vi "main.vi"(11 "Message Input":T1) -> (5 "Message Output":T1)   [LabVIEW 2025, in "Module 2.lvlib"]
uses:
  Module 2.lvlib
  <extravilib>/ChannelInstances/Event Messenger-t'Channel Messages.lvlib-Message Cluster.ctl'/))Channel.ctl
  Channel Messages/Message Cluster.ctl
  Module 2 Cases.ctl
  0fcfb8a4-f357-4310-b837-e68650746e25.vi
  <vilib>/Utility/error.llb/Clear Errors.vi
  <extravilib>/ChannelInstances/Event Messenger-t'Channel Messages.lvlib-Message Cluster.ctl'/))Channel.vi
  Channel Messages/9242 error converting cmd string to case enum--error.vi
  <extravilib>/ChannelInstances/Event Messenger-t'Channel Messages.lvlib-Message Cluster.ctl'.lvlib
  Channel Messages/Channel Messages.lvlib
panel:
  in  "Process Stop Button":bool
  in  "Record Button":bool
  out "Log":string
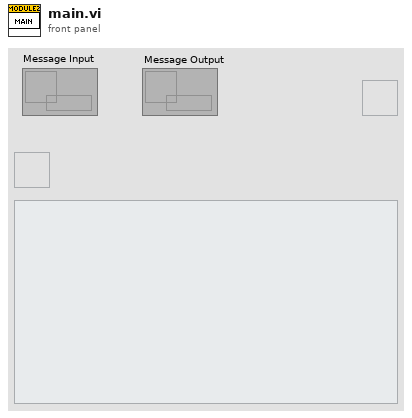
[diagram p1: front panel]
types:
  T1 = typedef "Event Messenger-t'Channel Messages.lvlib-Message Cluster.ctl'.lvlib/))Channel.ctl" = refnum<queue>
  T2 = typedef "Channel Messages.lvlib/Message Cluster.ctl" = cluster{"cmd":string, "data":variant}
  T3 = typedef "Module 2 Cases.ctl" = enum16{"Kill", "Stop", "Start", "Log"}
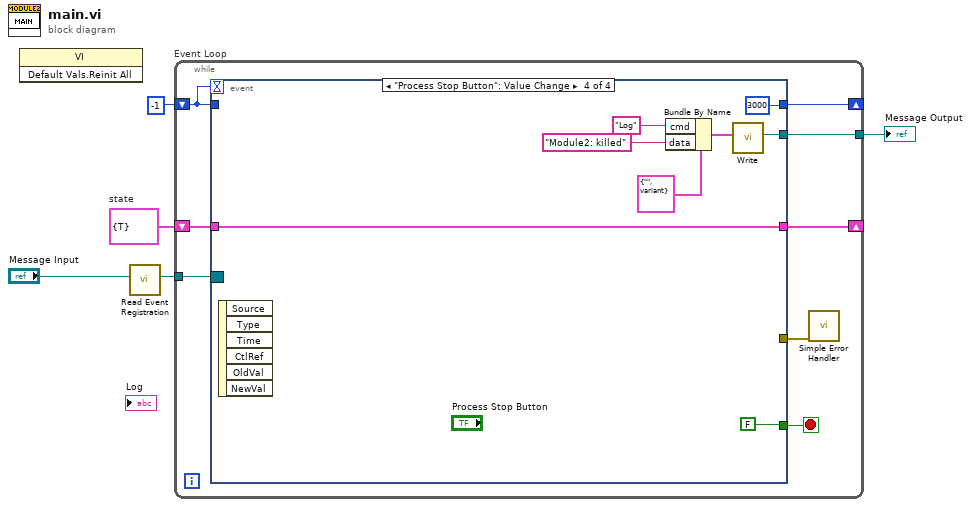
[diagram p0: block diagram]
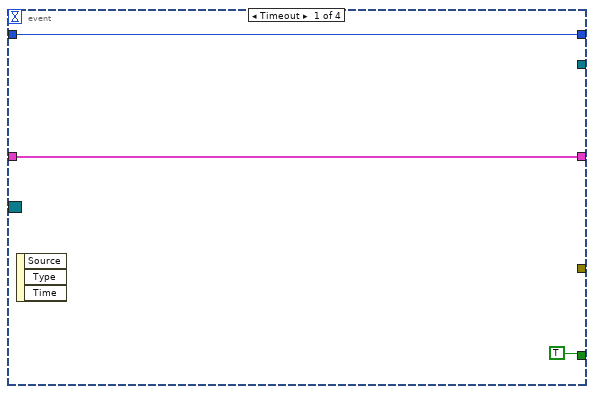
[diagram p2: hidden frame]
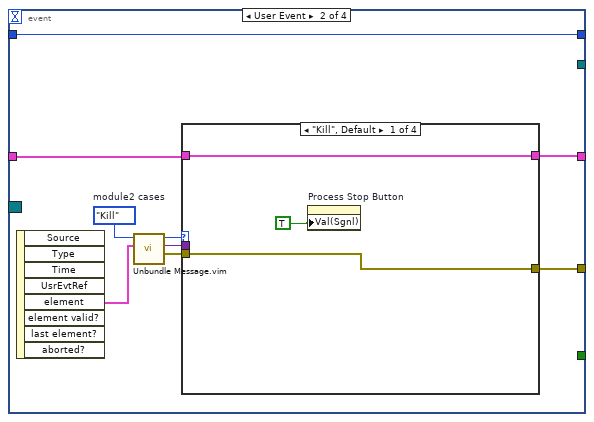
[diagram p3: hidden frame]
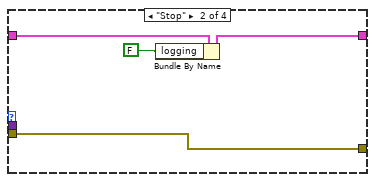
[diagram p4: hidden frame]
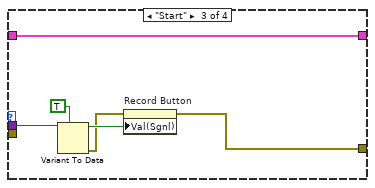
[diagram p5: hidden frame]
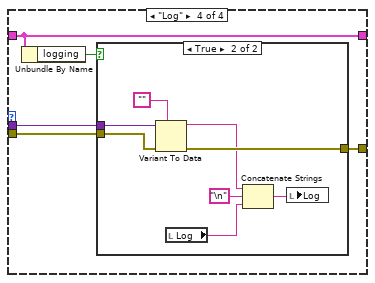
[diagram p6: hidden frame]
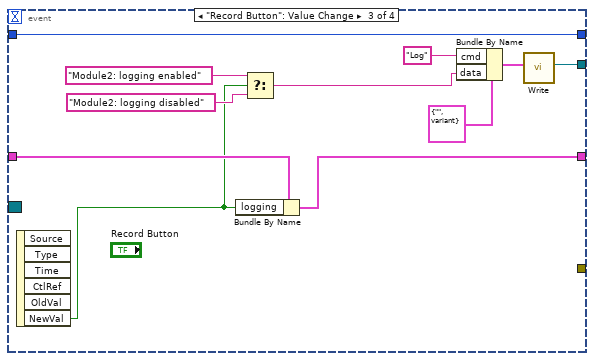
[diagram p8: hidden frame]
diagram:
  w5 = cluster{"logging":bool} {"logging"=TRUE}  # state
  n1 = invoke class="VI" method="Default Vals.Reinit All"() -> ()  [unwired: 3 in, 3 out]
  n2 = call <extravilib>:"Read Event Registration.vi"("channel"="Message Input") -> ("event registration refnum"=w3:refnum<event-registration>)  [unwired: 10 in]
  n3 = while "Event Loop" {
    shift-right: [w11] -> _
    shift-left: w5 -> [w12]
    tunnel: w3 -> [w9]
    tunnel: [w8] -> w2
    shift-right: [w6] -> _
    shift-left: -1 -> [w7]
    stop <- w13 stop-if-true
    n4 = event shown="[3] \"Process Stop Button\": Value Change" {
      selector: w9 -> [_ _ _ _]
      dyn-events: _ -> [_ _ _ _]
      timeout: w7 -> [_ _ _ _]
      tunnel: [TRUE _ _ FALSE] -> w13
      tunnel: w12 -> [w14 w22 w63 w64]
      tunnel: [w14 w21 w62 w64] -> w11
      tunnel: [_ w19 _ _] -> w10
      tunnel: [_ _ w57 w68] -> w8
      tunnel: w7 -> [w15 w17 w53 _]
      tunnel: [w15 w17 w53 3000] -> w6
      event Timeout {
        n5 = event-data() -> ()  [unwired: 1 in, 3 out]
      }
      event User Event {
        w24 = Module_2_Cases."Kill"  # module2 cases
        n6 = event-data() -> ("element"=w23:T2)  [unwired: 1 in, 7 out]
        n7 = call "Unbundle Message.vim"("message"=w23, "cases type"=w24) -> ("error out"=w20:errorcluster, "data"=w25:variant, "case"=w18:T3)  [unwired: 7 in]
        n8 = case shown="\"Kill\", Default" w18 {
          tunnel: w25 -> [_ _ w38 w41]
          tunnel: w22 -> [w28 w32 w33 w43]
          tunnel: [w28 w30 w33 w43] -> w21
          tunnel: [w27 w31 w34 w40] -> w19
          tunnel: w20 -> [w27 w31 _ w39]
          frame "Kill", Default {
            n9 = property on="Process Stop Button" class="Bool (strict)"("Val(Sgnl)"=TRUE ("Value (Signaling)")) -> ()  [unwired: 2 in, 2 out]
          }
          frame "Stop" {
            n10 = Bundle By Name(cluster=w32, "logging"=FALSE) -> (w30:cluster{"logging":bool})
          }
          frame "Start" {
            n11 = Variant To Data(type=TRUE, Variant=w38) -> (data=w36:bool, error out=w35:errorcluster)  [unwired: 1 in]
            n12 = property on="Record Button" class="Bool (strict)"(error in=w35, "Val(Sgnl)"=w36) -> (error out=w34:errorcluster)  [unwired: 1 in, 1 out]
          }
          frame "Log" {
            n13 = Unbundle By Name(w43) -> ("logging"=w42:bool)
            n14 = case shown="True" w42 {
              tunnel: w41 -> [_ w52]
              tunnel: [w44 w51] -> w40
              tunnel: w39 -> [w44 w45]
              frame False {
              }
              frame True {
                n15 = Variant To Data(error in=w45, type="", Variant=w52) -> (data=w47:string, error out=w51:errorcluster)
                n16 = local read "Log"() -> (w49:string)
                n17 = Concatenate Strings(w47, "\n", w49) -> (w48:string)
                n18 = local write "Log"(w48) -> ()
              }
            }
          }
        }
      }
      event "Record Button": Value Change {
        n19 = event-data() -> ("NewVal"=w54:bool)  [unwired: 1 in, 5 out]
        n20 = Bundle By Name(cluster=w63, "logging"=w54) -> (w62:cluster{"logging":bool})
        n21 = Select(t="Module2: logging enabled", s=w54, f="Module2: logging disabled") -> (s? t:f=w56:string)
        n22 = Bundle By Name(cluster=T2 {"cmd"="", "data"=variant} ("message"), "cmd"="Log", "data"=w56) -> (w58:T2)
        n23 = call <extravilib>:"Write.vi"("element"=w58) -> ("channel"=w57:T1)  [unwired: 9 in, 1 out]
      }
      event "Process Stop Button": Value Change {
        n24 = event-data() -> ()  [unwired: 1 in, 6 out]
        n25 = Bundle By Name(cluster=T2 {"cmd"="", "data"=variant} ("message"), "cmd"="Log", "data"="Module2: killed") -> (w69:T2)
        n26 = call <extravilib>:"Write.vi"("element"=w69) -> ("channel"=w68:T1)  [unwired: 9 in, 1 out]
      }
    }
    n27 = call <vilib>:"Simple Error Handler.vi"("error in (no error)"=w10) -> ()  [unwired: 4 in, 5 out]
  }
  "Message Output" <- w2
